vi "Disonnect Trigger Terminals.vi"(8 "error in (no error)":errorcluster, 10 "Routing Information":T1={"Source"="PXI_Trig0", "Destination"="PXI_Trig0", "Synchronization Clock"="SyncClkAsync"}, 11 "instrument handle":refnum<k15>) -> (0 "error out":errorcluster, 3 "instrument handle out":refnum<k15>)   [LabVIEW 2026]
doc: "This VI allows an array input of Trigger Routing Controls. NI-SYNC will make the connects of each array input. The benefit of this vi is there is no need for multiple string inputs."
uses:
  Trigger Routing.ctl
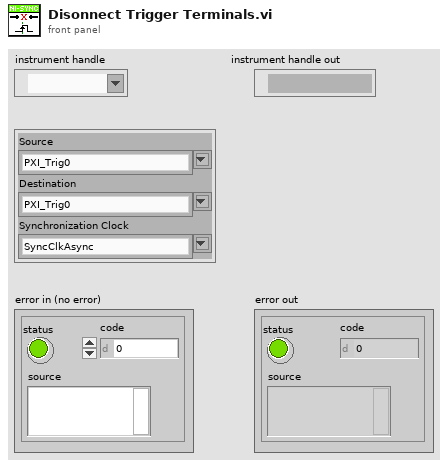
[diagram p1: front panel]
types:
  T1 = typedef "Trigger Routing.ctl" = cluster{"Source":string, "Destination":string, "Synchronization Clock":string}
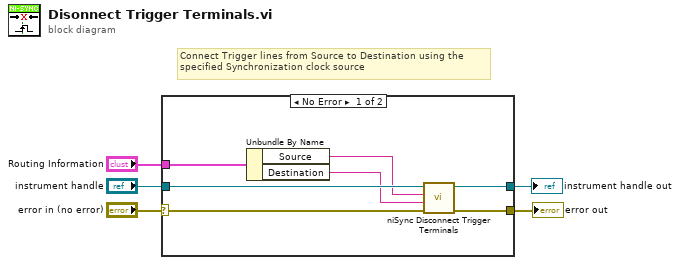
[diagram p0: block diagram]
diagram:
  # "Connect Trigger lines from Source to Destination using the\nspecified Synchronization clock source"
  n1 = case shown="No Error" "error in (no error)" {
    selector: "error in (no error)" -> [w9 w14]
    tunnel: "Routing Information" -> [w12 _]
    tunnel: "instrument handle" -> [w11 w13]
    tunnel: [w10 w13] -> w4
    tunnel: [w8 w14] -> w2
    frame No Error {
      n2 = Unbundle By Name(w12) -> ("Source"=w7:string, "Destination"=w6:string)
      n3 = call <instrlib>:"niSync Disconnect Trigger Terminals.vi"("error in (no error)"=w9, "destination terminal"=w6, "source terminal"=w7, "instrument handle"=w11) -> ("error out"=w8:errorcluster, "instrument handle out"=w10:refnum<k15>)  [unwired: 6 in]
    }
    frame Error {
    }
  }
  "instrument handle out" <- w4
  "error out" <- w2
